vi "doDFSM_Idle.vi"(0 "NInstrSim":refnum<class "NInstrSim.lvclass">, 3 "DFSM_Internals in":T1, 5 "error in (no error)":errorcluster) -> (14 "dup NInstrSim":refnum<class "NInstrSim.lvclass">, 17 "DFSM_Internals out":T1, 19 "error out":errorcluster)   [LabVIEW 2009, in "HB_Device_Examples.lvlib" / "NInstrSim.lvclass"]
doc: "This VI performs <B>do</B> action of DeviceFSM.Active.\n\n<b>Hint:</b> This is a dynamic dispatch VI to be implemented by child classes."
uses:
  NInstrSim.lvclass
  lib.lib/HGF_LVC/HGF_StateCharts/HGF_DeviceFSM/HGF_DeviceFSM_Internals.ctl
  lib.lib/HGF_LVC/HGF_DeviceBaseClasses/HGF_VISADevice/HGF_VISADevice.lvclass
  lib.lib/HGF_LVC/HGF_DeviceBaseClasses/HGF_DeviceBaseClasses.lvlib
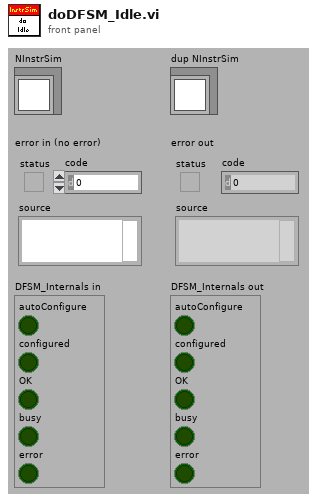
[diagram p1: front panel]
types:
  T1 = typedef "HGF_DeviceBaseClasses.lvlib/HGF_DeviceFSM_Internals.ctl" = cluster{"autoConfigure":bool, "configured":bool, "OK":bool, "busy":bool, "error":bool}
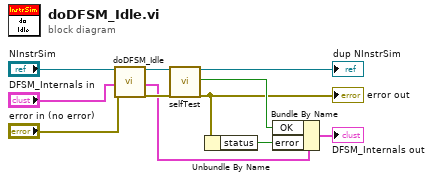
[diagram p0: block diagram]
diagram:
  n1 = call-parent "doDFSM_Idle.vi"("HGF_DeviceBase"="NInstrSim", "DFSM_Internals in"="DFSM_Internals in", "error in (no error)"="error in (no error)") -> ("dup HGF_DeviceBase"=w8:refnum<class "NInstrSim.lvclass">, "DFSM_Internals out"=w4:T1, "error out"=w6:errorcluster)  [unwired: 14 out]
  n2 = call-dynamic "selfTest.vi"("NInstrSim"=w8, "error in (no error)"=w6) -> ("dup NInstrSim"=→"dup NInstrSim":refnum<class "NInstrSim.lvclass">, "passed?"=w5:bool, "error out"=w2:errorcluster)  [unwired: 15 out]
  "error out" <- w2
  n3 = Unbundle By Name(w2) -> ("status"=w1:bool)
  n4 = Bundle By Name(cluster=w4, "OK"=w5, "error"=w1) -> (→"DFSM_Internals out":T1)
